vi "Timing Message Loop.vi"(8 "error in (no error)":errorcluster, 10 "Timers":T1, 11 "Message Queues":T2) -> (0 "error out":errorcluster)   [LabVIEW 2018, in "Message Queue.lvlib"]
uses:
  Message Queue.lvlib
  All Message Queues.ctl
  Message Cluster.ctl
  Acquisition/Acquisition State.ctl
  controls/ExitGlobal.vi
  Enqueue Message (Single).vi
  <vilib>/Utility/error.llb/Error Cluster From Error Code.vi
  <vilib>/ErrorRing/Error Ring.xnode
  Acquisition/Acquisition.lvlib
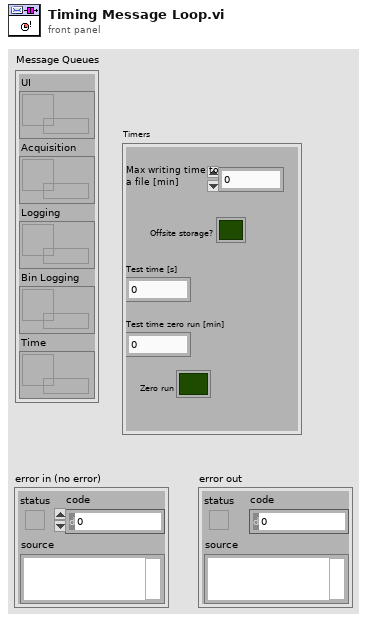
[diagram p1: front panel]
types:
  T1 = cluster{"Offsite storage?":bool, "Test time [s]":dbl, "Test time zero run [s] ":dbl, "Max writing time to a file [min]":dbl, "Zero run":bool}
  T2 = typedef "Message Queue.lvlib/All Message Queues.ctl" = cluster{"UI":refnum<queue>, "Acquisition":refnum<queue>, "Logging":refnum<queue>, "Bin Logging":refnum<queue>, "Time":refnum<queue>}
  T3 = typedef "Acquisition.lvlib/Acquisition State.ctl" = enum16{"Idle", "Acquiring"}
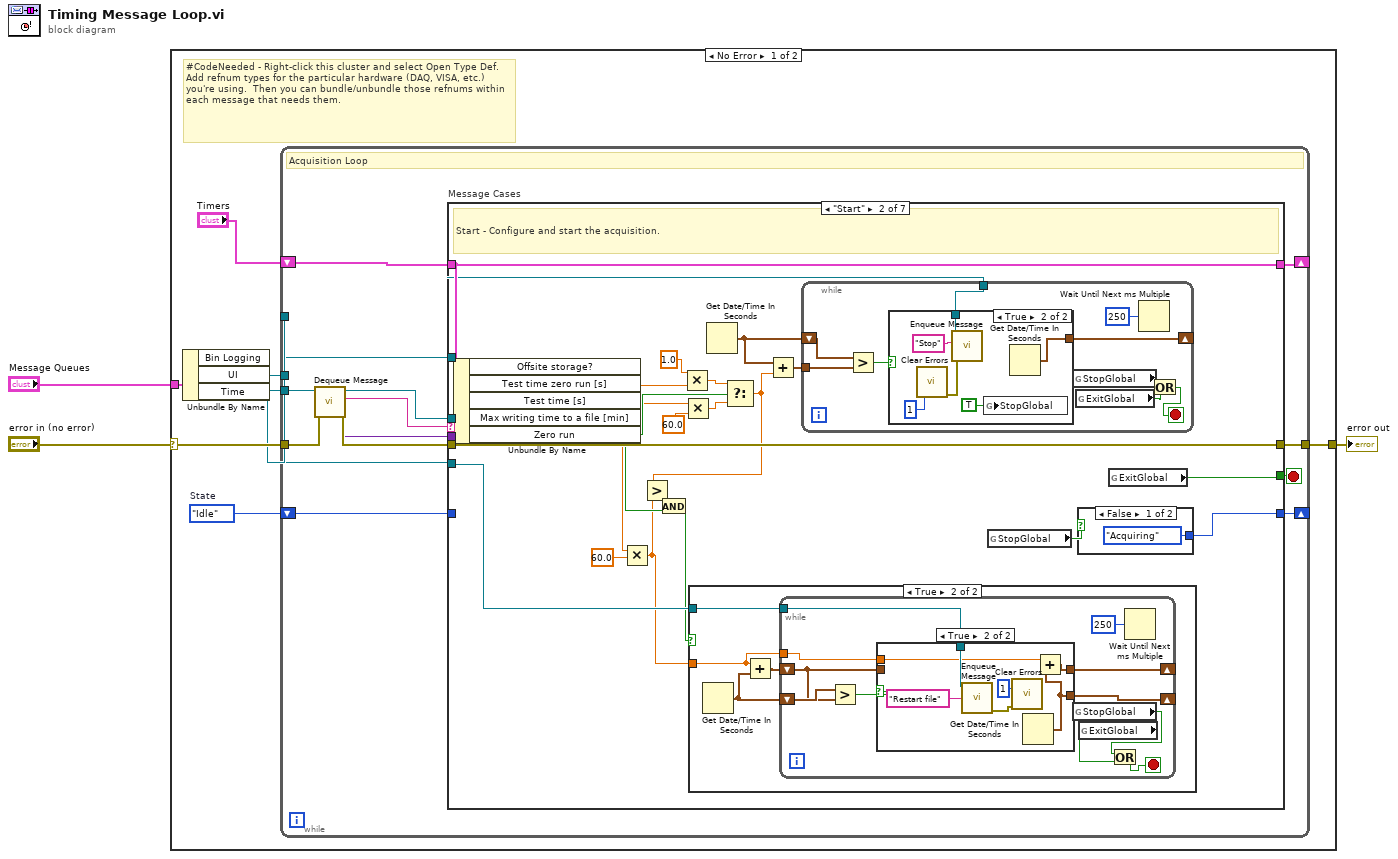
[diagram p0: block diagram]
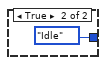
[diagram p3: hidden frame]
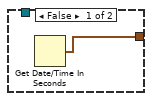
[diagram p4: hidden frame]
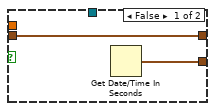
[diagram p6: hidden frame]
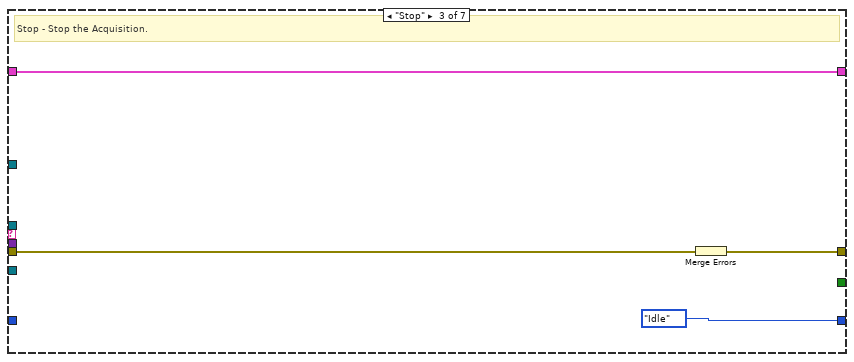
[diagram p7: hidden frame]
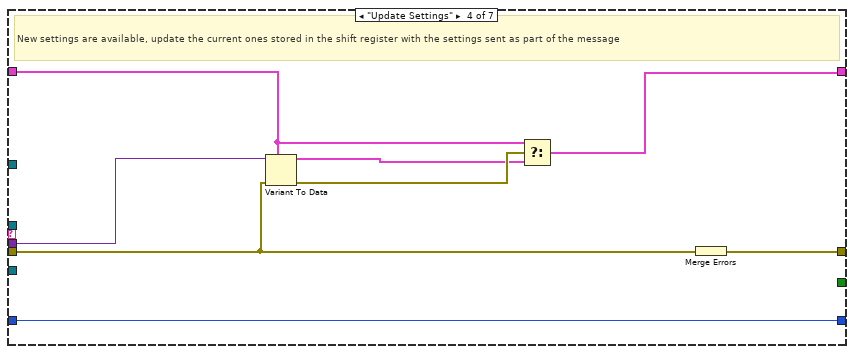
[diagram p8: hidden frame]
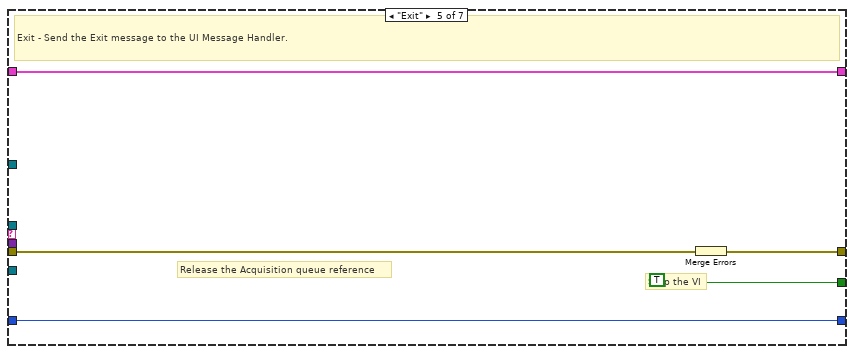
[diagram p9: hidden frame]
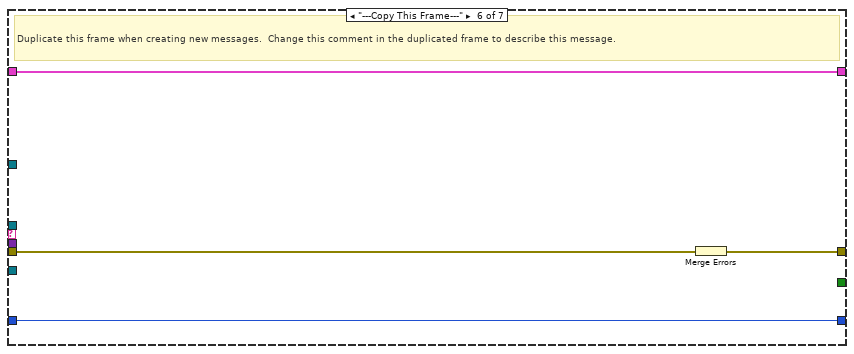
[diagram p10: hidden frame]
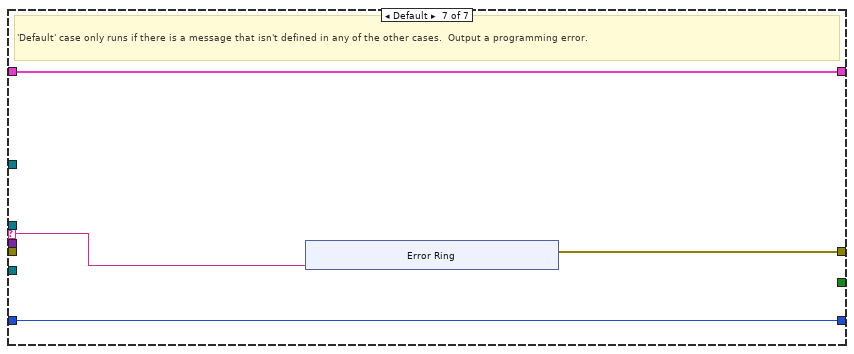
[diagram p11: hidden frame]
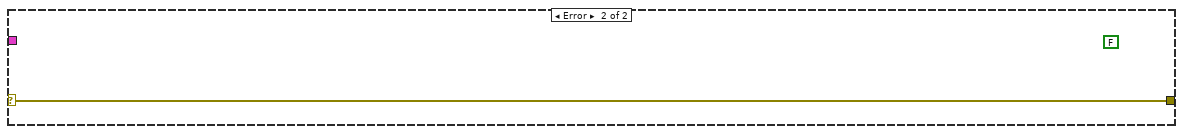
[diagram p12: hidden frame]
diagram:
  n1 = case shown="No Error" "error in (no error)" {
    selector: "error in (no error)" -> [w9 w126]
    tunnel: "Message Queues" -> [w11 _]
    tunnel: [w5 w126] -> w2
    frame No Error {
      w7 = Acquisition_State."Idle"  # State
      # "#CodeNeeded - Right-click this cluster and select Open Type Def.  Add refnum types for the particular hardware (DAQ, VISA, etc.) you're using.  Then you can bundle/unbundle those refnums within each message that needs them."
      n2 = Unbundle By Name(w11) -> ("Bin Logging"=w4:refnum<queue>, "UI"=w8:refnum<queue>, "Time"=w10:refnum<queue>)
      n3 = while {
        tunnel: w10 -> [w20]
        shift-right: [w24] -> _
        shift-left: "Timers" -> [w25]
        tunnel: w8 -> [w16]
        shift-right: [w18] -> _
        shift-left: w7 -> [w19]
        tunnel: w9 -> [w22]
        tunnel: [w15] -> w5
        tunnel: w4 -> [w14]
        stop <- w23 stop-if-true
        # "Acquisition Loop"
        n4 = call "Dequeue Message.vi"("error in (no error)"=w22, "Message Queue"=w20) -> ("error out"=w21:errorcluster, "Message Data"=w13:variant, "Message"=w12:string, "dup Message Queue"=w17:refnum<queue>)  [unwired: 6 in]
        n5 = case "Message Cases" shown="\"Start\"" w12 {
          selector: w12 -> [_ _ _ _ _ _ w115]
          tunnel: w17 -> [_ _ _ _ _ _ _]
          tunnel: w21 -> [w28 w51 w95 w101 w106 w114 _]
          tunnel: [w28 w51 w97 w105 w109 w112 w116] -> w15
          tunnel: w25 -> [w27 w49 w96 w98 w108 w113 w118]
          tunnel: [w27 w49 w96 w102 w108 w113 w118] -> w24
          tunnel: [_ w48 _ _ TRUE _ _] -> w23
          tunnel: w13 -> [_ _ _ w99 _ _ _]
          tunnel: w16 -> [_ w41 _ _ _ _ _]
          tunnel: w19 -> [w26 _ _ w100 w107 w111 w117]
          tunnel: [w26 w30 Acquisition_State."Idle" ("State") w100 w107 w111 w117] -> w18
          tunnel: w14 -> [_ w47 _ _ _ _ _]
          frame "Initialize" {
            # "Initialize  - Initialize is currently a no-op.  The hardware initialization takes place in the 'Start' message."
          }
          frame "Start" {
            # "Start - Configure and start the acquisition."
            n6 = Unbundle By Name(w49) -> ("Offsite storage?"=w42:bool, "Test time zero run [s]"=w35:dbl, "Test time [s]"=w39:dbl, "Max writing time to a file [min]"=w46:dbl, "Zero run"=w50:bool)
            n7 = Multiply(x=w46, y=60.0) -> (x*y=w31:dbl)
            n8 = Multiply(x=1.0 ("y"), y=w35) -> (x*y=w37:dbl)
            n9 = Multiply(x=w39, y=60.0) -> (x*y=w36:dbl)
            n10 = Get Date/Time In Seconds() -> (seconds since 1Jan1904=w32:timestamp)
            n11 = Select(t=w37, s=w50, f=w36) -> (s? t:f=w34:dbl)
            n12 = Greater?(x=w34, y=w31) -> (0:w43:bool)
            n13 = And(x=w43, y=w42) -> (x .and. y?=w44:bool)
            n14 = case shown="True" w44 {
              tunnel: w47 -> [_ w73]
              tunnel: w31 -> [_ w70]
              frame False {
              }
              frame True {
                n15 = Get Date/Time In Seconds() -> (seconds since 1Jan1904=w71:timestamp)
                n16 = Add(x=w70, y=w71) -> (x+y=w72:timestamp)
                n17 = while {
                  tunnel: w73 -> [w84]
                  shift-right: [w80] -> _
                  shift-left: w71 -> [w82]
                  shift-right: [w75] -> _
                  shift-left: w72 -> [w76]
                  tunnel: w70 -> [w74]
                  stop <- w77 stop-if-true
                  n18 = Greater?(x=w82, y=w76) -> (0:w81:bool)
                  n19 = case shown="True" w81 {
                    tunnel: w84 -> [_ w93]
                    tunnel: [w86 w89] -> w80
                    tunnel: w76 -> [w85 _]
                    tunnel: [w85 w88] -> w75
                    tunnel: w74 -> [_ w87]
                    frame False {
                      n20 = Get Date/Time In Seconds() -> (seconds since 1Jan1904=w86:timestamp)
                    }
                    frame True {
                      n21 = call-poly "Enqueue Message.vi"("Message"="Restart file" ("t"), "Message Queue"=w93) -> ("error out"=w92:errorcluster)  [unwired: 8 in, 1 out]
                      n22 = call <vilib>:"Clear Errors.vi"("error in (no error)"=w92, "specific error code to clear (0: all)"=1) -> ()  [unwired: 4 in, 2 out]
                      n23 = Get Date/Time In Seconds() -> (seconds since 1Jan1904=w89:timestamp)
                      n24 = Add(x=w87, y=w89) -> (x+y=w88:timestamp)
                    }
                  }
                  n25 = global read "ExitGlobal.vi" "StopGlobal"() -> (w79:bool)
                  n26 = global read "ExitGlobal.vi" "ExitGlobal"() -> (w78:bool)
                  n27 = Or(x=w79, y=w78) -> (x .or. y?=w77:bool)
                  n28 = Wait Until Next ms Multiple(millisecond multiple=u32 250) -> ()  [unwired: 1 out]
                }
              }
            }
            n29 = Add(x=w32, y=w34) -> (x+y=w33:timestamp)
            n30 = while {
              tunnel: w41 -> [w62]
              tunnel: w33 -> [w60]
              shift-right: [w57] -> _
              shift-left: w32 -> [w58]
              stop <- w54 stop-if-true
              n31 = Greater?(x=w58, y=w60) -> (0:w59:bool)
              n32 = case shown="True" w59 {
                tunnel: w62 -> [_ w69]
                tunnel: [w63 w65] -> w57
                frame False {
                  n33 = Get Date/Time In Seconds() -> (seconds since 1Jan1904=w63:timestamp)
                }
                frame True {
                  n34 = call-poly "Enqueue Message.vi"("Message"="Stop" ("value in"), "Message Queue"=w69) -> ("error out"=w67:errorcluster)  [unwired: 8 in, 1 out]
                  n35 = call <vilib>:"Clear Errors.vi"("error in (no error)"=w67, "specific error code to clear (0: all)"=1) -> ()  [unwired: 4 in, 2 out]
                  n36 = global write "ExitGlobal.vi" "StopGlobal"(TRUE ("StopGlobal")) -> ()
                  n37 = Get Date/Time In Seconds() -> (seconds since 1Jan1904=w65:timestamp)
                }
              }
              n38 = global read "ExitGlobal.vi" "StopGlobal"() -> (w56:bool)
              n39 = global read "ExitGlobal.vi" "ExitGlobal"() -> (w55:bool)
              n40 = Wait Until Next ms Multiple(millisecond multiple=u32 250) -> ()  [unwired: 1 out]
              n41 = Or(x=w56, y=w55) -> (x .or. y?=w54:bool)
            }
            n42 = global read "ExitGlobal.vi" "StopGlobal"() -> (w29:bool)
            n43 = case shown="False" w29 {
              tunnel: [Acquisition_State."Acquiring" ("State") Acquisition_State."Idle" ("State")] -> w30
              frame False {
              }
              frame True {
              }
            }
            n44 = global read "ExitGlobal.vi" "ExitGlobal"() -> (w48:bool)
          }
          frame "Stop" {
            # "Stop - Stop the Acquisition."
            n45 = Merge Errors(w95) -> (w97:errorcluster)
          }
          frame "Update Settings" {
            # "New settings are available, update the current ones stored in the shift register with the settings sent as part of the message"
            n46 = Variant To Data(error in=w101, type=w98, Variant=w99) -> (data=w103:T1, error out=w104:errorcluster)
            n47 = Select(t=w98, s=w104, f=w103) -> (s? t:f=w102:T1)
            n48 = Merge Errors(w101) -> (w105:errorcluster)
          }
          frame "Exit" {
            # "Release the Acquisition queue reference"
            # "Stop the VI"
            # "Exit - Send the Exit message to the UI Message Handler."
            n49 = Merge Errors(w106) -> (w109:errorcluster)
          }
          frame "---Copy This Frame---" {
            # "Duplicate this frame when creating new messages.  Change this comment in the duplicated frame to describe this message."
            n50 = Merge Errors(w114) -> (w112:errorcluster)
          }
          frame Default {
            # "'Default' case only runs if there is a message that isn't defined in any of the other cases.  Output a programming error."
            n51 = xnode "Error Ring"("parameter 0"=w115) -> ("error out"=w116:errorcluster)
          }
        }
      }
    }
    frame Error {
      (unwired) FALSE ("Running")
    }
  }
  "error out" <- w2
